vi "DriveBase.vi"(9 "Elevator State":string="Hatch_Rocket_1") -> ()   [LabVIEW 2018]
uses:
  RobotStates.vi
  Inputs_DriverStation.vi
  SensorReadings.vi
panel:
  in  "Elevator Danger Height (in)":dbl=100.0
  in  "Max Acceleration (power/s)":dbl=3.0
  in  "Climb-Drive Bias":dbl=-0.1
  in  "Turning Deadband":dbl=0.1
  in  "Throttle Deadband":dbl=0.1
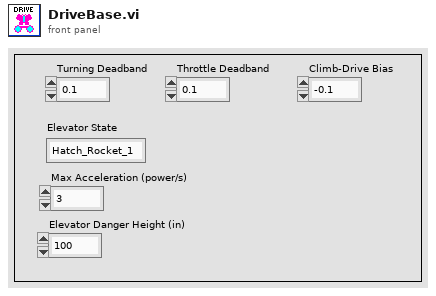
[diagram p1: front panel]
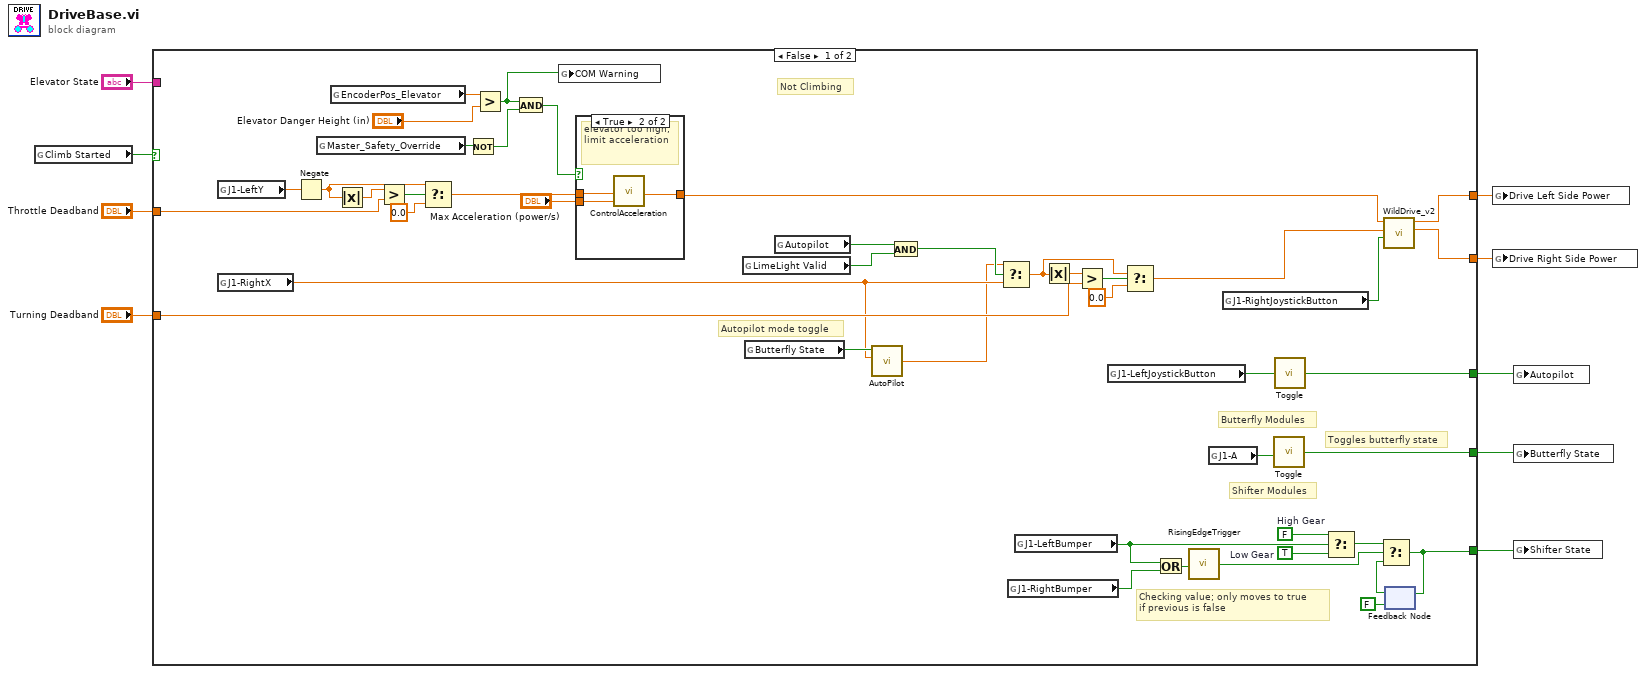
[diagram p0: block diagram]
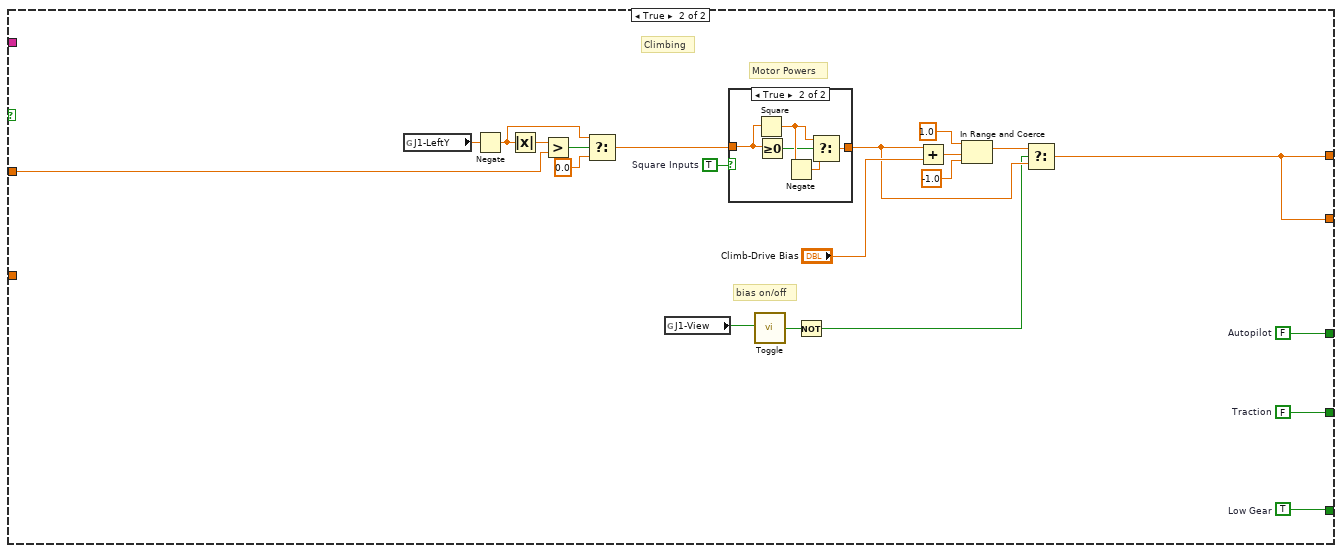
[diagram p3: hidden frame]
diagram:
  n1 = global read "RobotStates.vi" "Climb Started"() -> (w5:bool)
  n2 = case shown="False" w5 {
    tunnel: [w43 w69] -> w9
    tunnel: [w37 w78] -> w8
    tunnel: "Throttle Deadband" -> [w42 w70]
    tunnel: "Turning Deadband" -> [w41 _]
    tunnel: [w30 w59] -> w4
    tunnel: [w29 w59] -> w3
    tunnel: [w24 w58] -> w2
    tunnel: "Elevator State" -> [_ _]
    frame False {
      w32 = TRUE  # Low Gear
      w33 = FALSE  # High Gear
      # "Not Climbing"
      # "Autopilot mode toggle"
      # "Checking value; only moves to true \nif previous is false"
      # "Toggles butterfly state"
      # "Shifter Modules"
      # "Butterfly Modules"
      n3 = global read "Inputs_DriverStation.vi" "J1-LeftY"() -> (w49:dbl)
      n4 = global read "Inputs_DriverStation.vi" "J1-RightX"() -> (w12:dbl)
      n5 = Negate(x=w49) -> (-x=w52:dbl)
      n6 = global read "Inputs_DriverStation.vi" "Master_Safety_Override"() -> (w15:bool)
      n7 = global read "SensorReadings.vi" "EncoderPos_Elevator"() -> (w18:dbl)
      n8 = Absolute Value(x=w52) -> (abs(x)=w47:dbl)
      n9 = Greater?(x=w47, y=w42) -> (0:w48:bool)
      n10 = Select(t=w52, s=w48, f=0.0) -> (s? t:f=w21:dbl)
      n11 = Not(x=w15) -> (.not. x?=w14:bool)
      n12 = Greater?(x=w18, y="Elevator Danger Height (in)") -> (0:w10:bool)
      n13 = And(x=w10, y=w14) -> (x .and. y?=w16:bool)
      n14 = global write "RobotStates.vi" "COM Warning"(w10) -> ()
      n15 = case shown="True" w16 {
        tunnel: w21 -> [w54 w57]
        tunnel: [w54 w56] -> w20
        tunnel: "Max Acceleration (power/s)" -> [_ w55]
        frame False {
          # "elevator down"
        }
        frame True {
          # "elevator too high, limit acceleration"
          n16 = call "ControlAcceleration.vi"("Max Acceleration (power/s)"=w55, "Raw"=w57) -> ("Controlled"=w56:dbl)  [unwired: 1 in]
        }
      }
      n17 = global read "SensorReadings.vi" "LimeLight Valid"() -> (w22:bool)
      n18 = global read "RobotStates.vi" "Butterfly State"() -> (w13:bool)
      n19 = global read "RobotStates.vi" "Autopilot"() -> (w26:bool)
      n20 = call "AutoPilot.vi"("human contribution"=w12, "State"=w13) -> ("End Contribution"=w11:dbl)  [unwired: 2 in]
      n21 = And(x=w26, y=w22) -> (x .and. y?=w23:bool)
      n22 = Select(t=w11, s=w23, f=w12) -> (s? t:f=w27:dbl)
      n23 = global read "Inputs_DriverStation.vi" "J1-RightBumper"() -> (w39:bool)
      n24 = global read "Inputs_DriverStation.vi" "J1-LeftBumper"() -> (w35:bool)
      n25 = Absolute Value(x=w27) -> (abs(x)=w50:dbl)
      n26 = Greater?(x=w50, y=w41) -> (0:w51:bool)
      n27 = global read "Inputs_DriverStation.vi" "J1-LeftJoystickButton"() -> (w25:bool)
      n28 = Select(t=w27, s=w51, f=0.0) -> (s? t:f=w53:dbl)
      n29 = Or(x=w35, y=w39) -> (x .or. y?=w40:bool)
      n30 = call "RisingEdgeTrigger.vi"("Raw Signal"=w40) -> ("Trigger"=w34:bool)
      n31 = global read "Inputs_DriverStation.vi" "J1-A"() -> (w44:bool)
      n32 = global read "Inputs_DriverStation.vi" "J1-RightJoystickButton"() -> (w28:bool)
      n33 = call "Toggle.vi"("Trigger"=w44) -> ("New Mode"=w43:bool)
      n34 = call "Toggle.vi"("Trigger"=w25) -> ("New Mode"=w24:bool)
      n35 = Select(t=w33, s=w35, f=w32) -> (s? t:f=w36:bool)
      n36 = call "WildDrive_v2.vi"("Super_Turn"=w28, "Turn"=w53, "Speed"=w20) -> ("Right Side Power"=w29:dbl, "Left Side Power"=w30:dbl)  [unwired: 7 in]
      n37 = feedback #1(FALSE ("Low Gear")) -> (w38:bool)
      n38 = Select(t=w36, s=w34, f=w38) -> (s? t:f=w37:bool)
      n39 = feedback-in #1(w37) -> ()
    }
    frame True {
      w58 = FALSE  # Autopilot
      w72 = TRUE  # Square Inputs
      w78 = TRUE  # Low Gear
      w69 = FALSE  # Traction
      # "Climbing"
      # "bias on/off"
      # "Motor Powers"
      n40 = global read "Inputs_DriverStation.vi" "J1-LeftY"() -> (w75:dbl)
      n41 = Negate(x=w75) -> (-x=w76:dbl)
      n42 = Absolute Value(x=w76) -> (abs(x)=w73:dbl)
      n43 = Greater?(x=w73, y=w70) -> (0:w74:bool)
      n44 = Select(t=w76, s=w74, f=0.0) -> (s? t:f=w77:dbl)
      n45 = global read "Inputs_DriverStation.vi" "J1-View"() -> (w64:bool)
      n46 = case shown="True" w72 {
        tunnel: [w79 w84] -> w61
        tunnel: w77 -> [w79 w83]
        frame False {
        }
        frame True {
          n47 = Square(x=w83) -> (x^2=w81:dbl)
          n48 = Greater Or Equal To 0?(x=w83) -> (x >= 0?=w80:bool)
          n49 = Negate(x=w81) -> (-x=w82:dbl)
          n50 = Select(t=w81, s=w80, f=w82) -> (s? t:f=w84:dbl)
        }
      }
      n51 = call "Toggle.vi"("Trigger"=w64) -> ("New Mode"=w63:bool)
      n52 = Not(x=w63) -> (.not. x?=w60:bool)
      n53 = Add(x=w61, y="Climb-Drive Bias") -> (x+y=w68:dbl)
      n54 = In Range and Coerce(upper limit=1.0, x=w68, lower limit=-1.0) -> (coerced(x)=w62:dbl)  [unwired: 1 out]
      n55 = Select(t=w62, s=w60, f=w61) -> (s? t:f=w59:dbl)
    }
  }
  n56 = global write "RobotStates.vi" "Drive Left Side Power"(w4) -> ()
  n57 = global write "RobotStates.vi" "Drive Right Side Power"(w3) -> ()
  n58 = global write "RobotStates.vi" "Autopilot"(w2) -> ()
  n59 = global write "RobotStates.vi" "Butterfly State"(w9) -> ()
  n60 = global write "RobotStates.vi" "Shifter State"(w8) -> ()
